vi "CALC_MARK_X_DATA.vi"(0 "VISA IN":refnum<visa-resource-name>, 1 "Marker number":i32, 5 "error in":errorcluster, 7 "Channel":i32) -> (14 "VISA Out":refnum<visa-resource-name>, 15 "X Axis":dbl, 19 "error out":errorcluster)   [LabVIEW 2018, in "PNA-X.lvlib"]
doc: "CALCulate<cnum>:MARKer<mkr>:Y? \n(Read-only) Reads the marker's Y-axis value. The format of the value depends on the current \nCALC:MARKER:FORMAT setting. If the marker is set as delta, the data is relative to the reference \nmarker. \n*Critical Note:\nA measurement must be active prior to using the Marker functions\nThe query always returns two numbers: \nSmith and Polar formats - (Real, Imaginary) \nLINPhase and LOGPhase - (Real, Imaginary) \nAll other formats - (Value,0) \nNote: To accurately read the marker Y-axis value with trace smoothing applied, the requested format \nmust match the displayed format. Otherwise, the returned value is un-smoothed data. For example, to \nread the smoothed marker value when measuring group delay, both the display format and the marker \nformat must be set to (Group) Delay. \nSee Critical Note \nParameters \n<cnum> Channel number of the measurement. There must be a selected measurement \non that channel. If unspecified, <cnum> is set to 1. \n<mkr> Any marker number from 1 to 10; if unspecified, value is set to 1. \nExamples CALC:MARK:Y? \ncalculate2:marker3:y? \nQuery Syntax CALCulate<cnum>:MARKer<mkr>:Y? \nReturn Type Numeric \nDefault Not applicable \nLast modified: \nMarch 27, 2007 Corrected Set? \nDec. 4, 2006 Added smoothing note to Y? \n1543\n\nCalculate:Math Commands \nControls math operations on the currently selected measurement and memory. \nClick on a blue keyword to view the command details. \nSee Also \nExample Programs \nLearn about Math Operations \nSynchronizing the PNA and Controller \nSCPI Command Tree \nCritical Note: CALCulate commands act on the selected measurement. You can select one \nmeasurement for each channel using Calc:Par:Select"
uses:
  PNA-X.lvlib
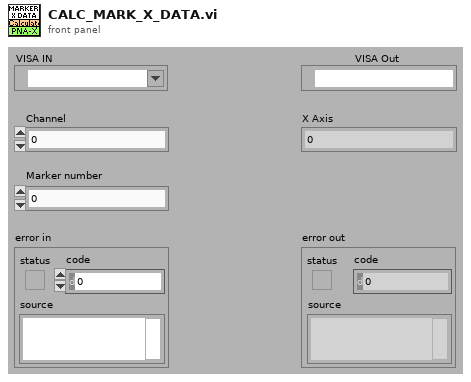
[diagram p1: front panel]
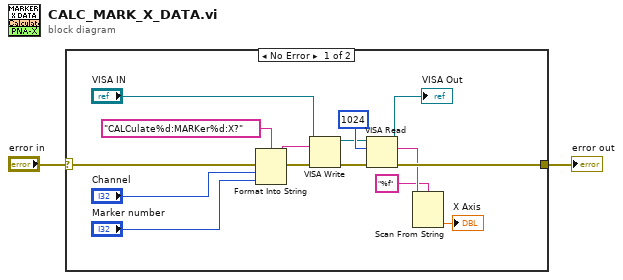
[diagram p0: block diagram]
diagram:
  n1 = case shown="No Error" "error in" {
    selector: "error in" -> [w17 w18]
    tunnel: [w9 w18] -> w1
    frame No Error {
      n2 = Format Into String(format string="CALCulate%d:MARKer%d:X?" ("Cmdline"), error in=w17, "Channel", "Marker number") -> (resulting string=w15:string, error out=w16:errorcluster)  [unwired: 1 in]
      n3 = VISA Write(VISA resource name="VISA IN", write buffer=w15, error in (no error)=w16) -> (VISA resource name out=w10:refnum<visa-resource-name>, error out=w12:errorcluster)  [unwired: 1 out]
      n4 = VISA Read(VISA resource name=w10, byte count=u32 1024, error in (no error)=w12) -> (VISA resource name out=→"VISA Out":refnum<visa-resource-name>, read buffer=w5:string, error out=w9:errorcluster)  [unwired: 1 out]
      n5 = Scan From String(format string="%f", input string=w5) -> (output 1=→"X Axis":dbl)  [unwired: 3 in, 3 out]
    }
    frame Error {
    }
  }
  "error out" <- w1
